vi "Calculate Voltage Deviation.vi"(10 "Nominal output voltage":dbl, 11 "Voltage measurements":dbl[](array[numeric])) -> (3 "Load voltage deviation":dbl[](array[numeric]))   [LabVIEW 2024]
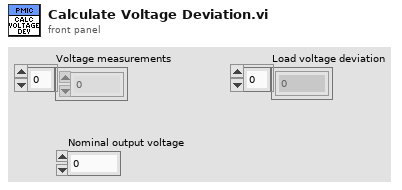
[diagram p1: front panel]
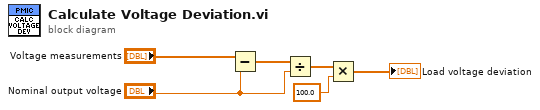
[diagram p0: block diagram]
diagram:
  n1 = Subtract(x="Voltage measurements", y="Nominal output voltage") -> (x-y=w3:dbl[])
  n2 = Divide(x=w3, y="Nominal output voltage") -> (x/y=w5:dbl[])
  n3 = Multiply(x=w5, y=100.0) -> (x*y=→"Load voltage deviation":dbl[])
